vi "Configure Trigger (Or).vi"(8 "error in (no error)":errorcluster, 10 "Or Edge Trigger (XXXXXXXXXXXXXXXXXX)":string="XXXXXXXXXXXXXXXXXX", 11 "VISA resource name":refnum<visa-resource-name>) -> (0 "error out":errorcluster, 3 "VISA resource name out":refnum<visa-resource-name>)   [LabVIEW 2019, in "Agilent 2000 3000 X-Series.lvlib"]
doc: "Configures the Or trigger mode."
uses:
  Agilent 2000 3000 X-Series.lvlib
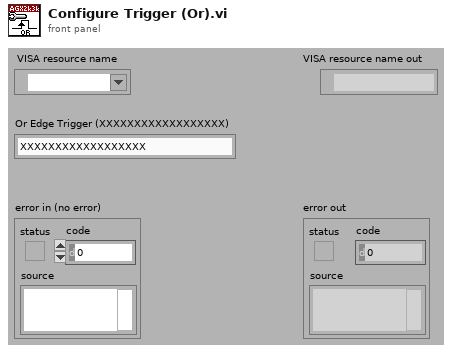
[diagram p1: front panel]
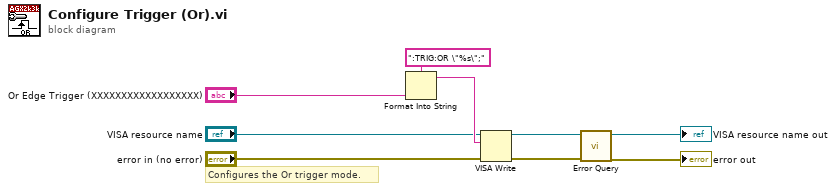
[diagram p0: block diagram]
diagram:
  # "Configures the Or trigger mode."
  n1 = Format Into String(format string=":TRIG:OR \"%s\";", "Or Edge Trigger (XXXXXXXXXXXXXXXXXX)") -> (resulting string=w7:string)  [unwired: 2 in, 1 out]
  n2 = VISA Write(VISA resource name="VISA resource name", write buffer=w7, error in (no error)="error in (no error)") -> (VISA resource name out=w4:refnum<visa-resource-name>, error out=w3:errorcluster)  [unwired: 1 out]
  n3 = call "Error Query.vi"("error in (no error)"=w3, "VISA resource name"=w4) -> ("error out"=→"error out":errorcluster, "VISA resource name out"=→"VISA resource name out":refnum<visa-resource-name>)  [unwired: 8 out]
